vi "Generate Publisher Message Set.vi"(9 "Mediator Enqueuer":refnum<class "Message Enqueuer.lvclass">, 11 "IMediator in":refnum<class "IMediator.lvclass">) -> (1 "Unlock Publication Msg":refnum<class "Unlock Publication Msg.lvclass">, 2 "Lock Publication Msg":refnum<class "Lock Publication Msg.lvclass">, 3 "Publish Msg":refnum<class "Publish Msg.lvclass">)   [LabVIEW 2019, in "IMediator.lvlib" / "IMediator.lvclass"]
uses:
  <vilib>/gpm_packages/@cs/mva-core/Source/IMediator/IMediator/IMediator.lvclass
  <vilib>/gpm_packages/@cs/mva-core/Source/IMediator/IMediator Messages/Publish Msg/Publish Msg.lvclass
  C:/Program Files/National Instruments/LabVIEW 2019/vi.lib/gpm_packages/@cs/actor-framework-messages/Source/RoundTripMessage/RoundTripMessage.lvclass
  <vilib>/gpm_packages/@cs/mva-core/Source/IMediator/IMediator Messages/Lock Publication Msg/Lock Publication Msg.lvclass
  <vilib>/gpm_packages/@cs/mva-core/Source/IMediator/IMediator Messages/Unlock Publication Msg/Unlock Publication Msg.lvclass
  <vilib>/ActorFramework/Message Enqueuer/Message Enqueuer.lvclass
  <vilib>/gpm_packages/@cs/actor-framework-messages/Source/RoundTripMessage/RoundTripMessage.lvclass/RoundTripMessage.ctl
  <vilib>/gpm_packages/@cs/actor-framework-messages/Source/RoundTripMessage/Write Return Address.vi
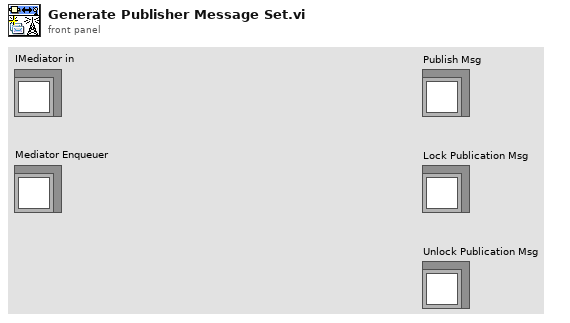
[diagram p1: front panel]
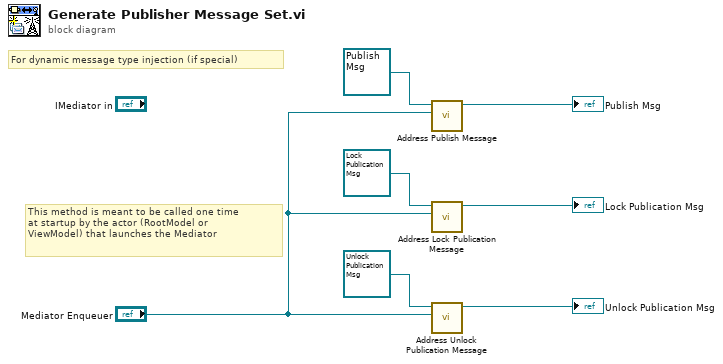
[diagram p0: block diagram]
diagram:
  # "This method is meant to be called one time\nat startup by the actor (RootModel or\nViewModel) that launches the Mediator"
  # "For dynamic message type injection (if special)"
  n1 = call <vilib>:"Address Publish Message.vi"("Mediator Enqueuer"="Mediator Enqueuer", "Publish Msg in"=refnum<class "Publish Msg.lvclass"> refnum ("Subscribe Msg In")) -> ("Publish Msg out"=→"Publish Msg":refnum<class "Publish Msg.lvclass">)  [unwired: 9 in]
  n2 = call <vilib>:"Address Lock Publication Message.vi"("Mediator Enqueuer"="Mediator Enqueuer", "Lock Publication Msg In"=refnum<class "Lock Publication Msg.lvclass"> refnum ("Unsubscribe Msg In")) -> ("Lock Publication Msg Out"=→"Lock Publication Msg":refnum<class "Lock Publication Msg.lvclass">)  [unwired: 9 in]
  n3 = call <vilib>:"Address Unlock Publication Message.vi"("Mediator Enqueuer"="Mediator Enqueuer", "Unlock Publication Msg In"=refnum<class "Unlock Publication Msg.lvclass"> refnum ("Unsubscribe Msg In")) -> ("Unlock Publication Msg Out"=→"Unlock Publication Msg":refnum<class "Unlock Publication Msg.lvclass">)  [unwired: 9 in]
